vi "SRC_var_globale.vi"() -> ()   [LabVIEW 2010, in "lv_04.lvlib"]
uses:
  lv_04.lvlib
panel:
  in  "Nb décimales":u16=2
  in  "Code src":string="004"
  in  "Chemin TDMS":path=path "D:/nidev/builds/lv_04/src_2.tdms"
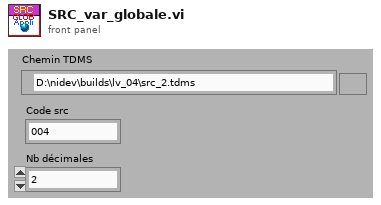
[diagram p1: front panel]
diagram:
